vi "status_parser.vi"(4 "error in (no error)":errorcluster, 6 "Motor #":u8) -> (0 "error out":errorcluster, 1 "Program Complete?":bool, 2 "Motor # dup":u8)   [LabVIEW 2015]
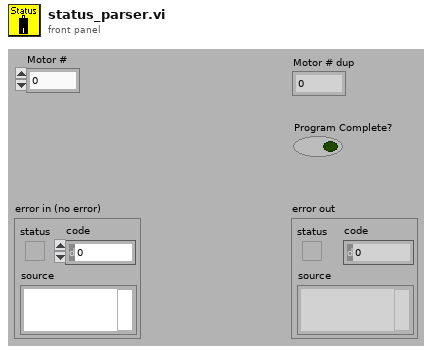
[diagram p1: front panel]
types:
  T1 = enum16{"POL (0)", "CPL (1)", "HLT (2)", "STP (3)", "RST (4)", "RVN (5)", "RPB (6)", "CLP (8)", "SDL (9)", "RUN (10)", "WRI (11)", "RRG (12)", "SPR (13)", "LPR (14)", "VMI (15)", "SSP (17)", "SSE (18)", "RIS (20)", "RIO (21)", "IMW (25)", "END (128)", "MAV (134)", "MRV (135)", "JRE (137)", "WCL (138)", "WCW (139)", "DLY (140)", "WDL (141)", "GCL (142)", "GOP (143)", "ZTG (144)", "ZTP (145)", "TTP (146)", "CME (147)", "CTC (148)", "TQL (149)", "AHC (150)", "ERL (151)", "OLP (152)", "WRP (154)", "IDT (155)", "LRP (156)", "VMP (159)", "RAV (160)", "RRV (161)", "JMP (162)", "JOI (162)", "CIS (163)", "CKS (164)", "CLC (165)", "KMC (167)", "MCT (168)", "FLC (169)", "EEM (170)", "DDB (171)", "DEM (171)", "PAC (172)", "ADL (173)", "BRT (174)", "MAT (176)", "MRT (177)", "RAT (178)", "RRT (179)", "SSD (180)", "KMR (181)", "KED (182)", "KDD (183)", "DIR (184)", "PRO (185)", "SIF (186)", "EDL (187)", "CIO (188)", "MDS (189)", "MDC (190)", "MDT (191)", "SEE (192)", "ARI (193)", "WBS (194)", "SCF (195)", "RSM (196)", "RLM (197)", "RSN (198)", "RLN (199)", "PCL (201)", "PCI (201)", "PRT (202)", "PRI (202)", "WBE (204)", "SOB (205)", "COB (206)", "ACR (207)", "PLR (208)", "CAI (211)", "LVT (212)", "OVT (213)", "MTT (214)", "CLC (215)", "PIM (216)", "VIM (217)", "TIM (218)", "AHM (219)", "SSL (221)", "TRU (222)", "RSD (223)", "EMT (225)", "DMT (226)", "EMD (227)", "DMD (228)", "HSM (229)", "AHD (230)", "PCM (231)", "PCG (232)", "XRV (233)", "XAV (234)", "XRT (235)", "XAT (236)", "GOC (237)", "JNA (238)", "JOR (239)", "PMC (240)", "PMV (241)", "PMX (242)", "DLC (243)", "SLC (244)", "PCP (245)", "ATR (248)", "PMO (249)", "JAN (250)", "EDH (251)", "DIF (252)", "IMS (253)", "IMQ (254)"}
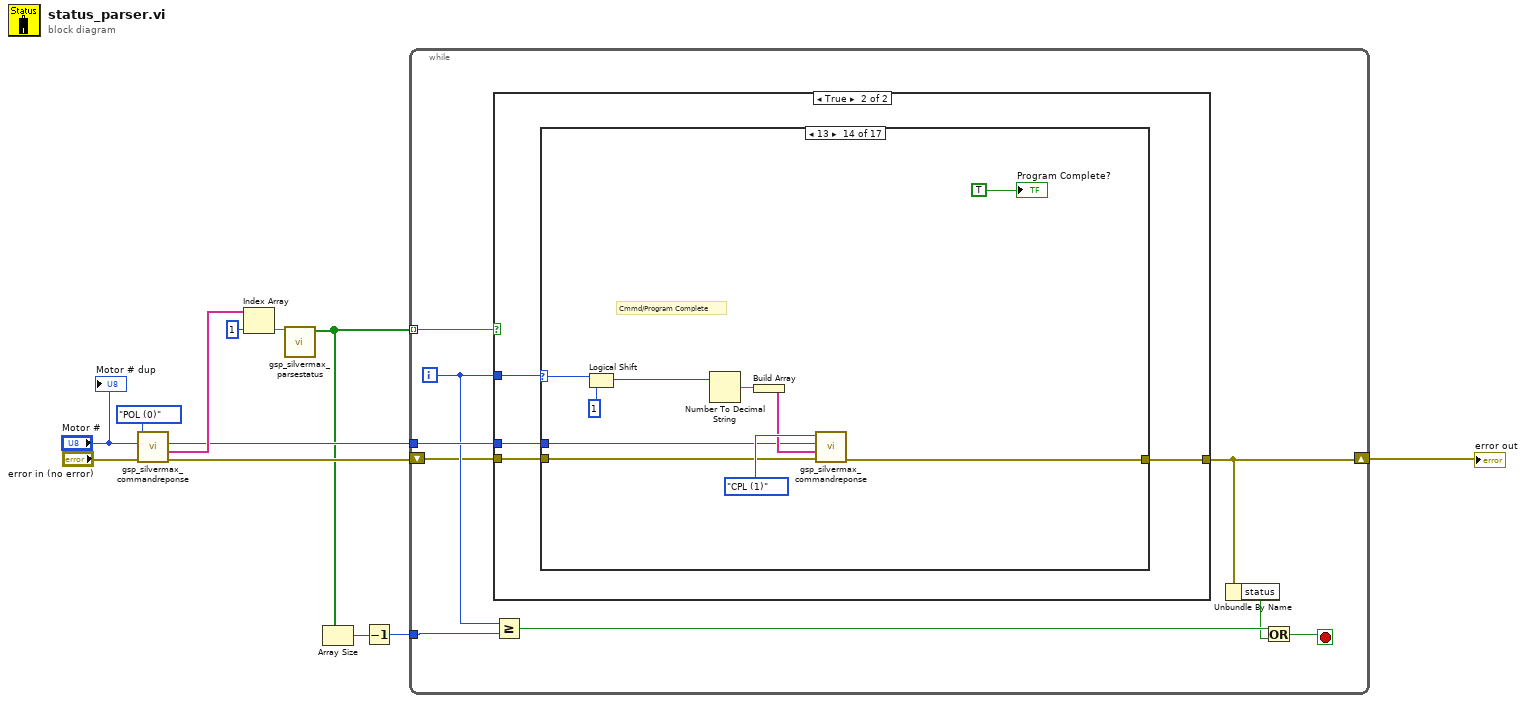
[diagram p0: block diagram]
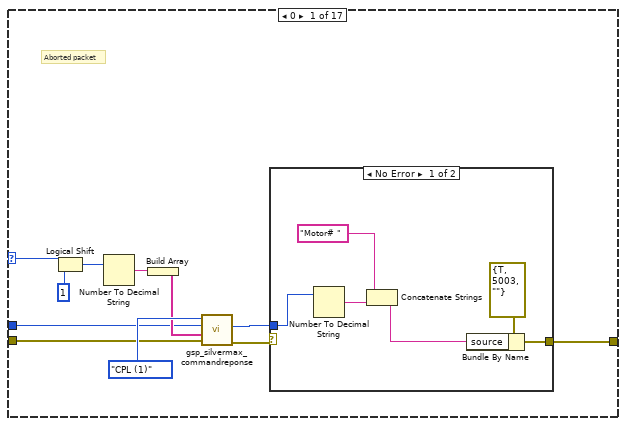
[diagram p3: hidden frame]
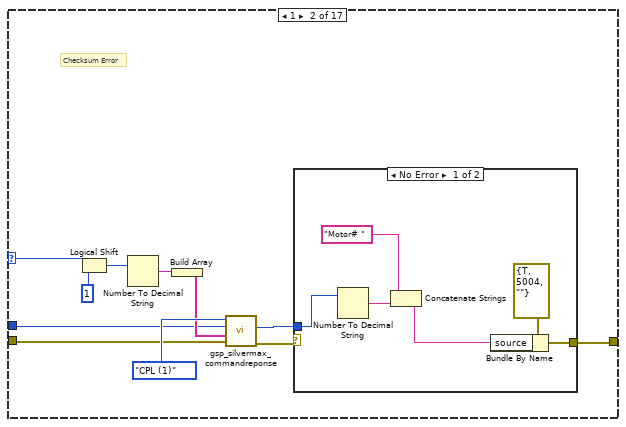
[diagram p5: hidden frame]
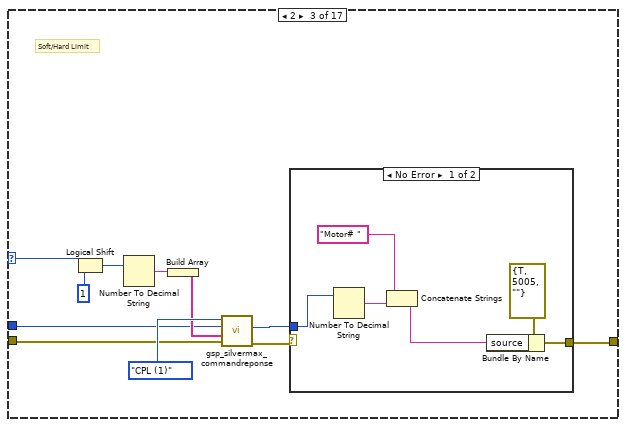
[diagram p7: hidden frame]
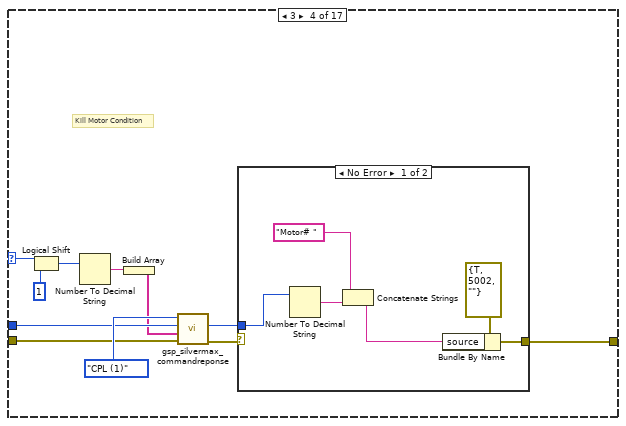
[diagram p9: hidden frame]
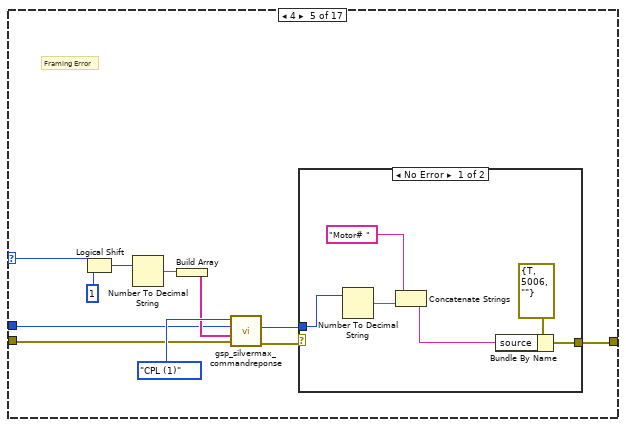
[diagram p11: hidden frame]
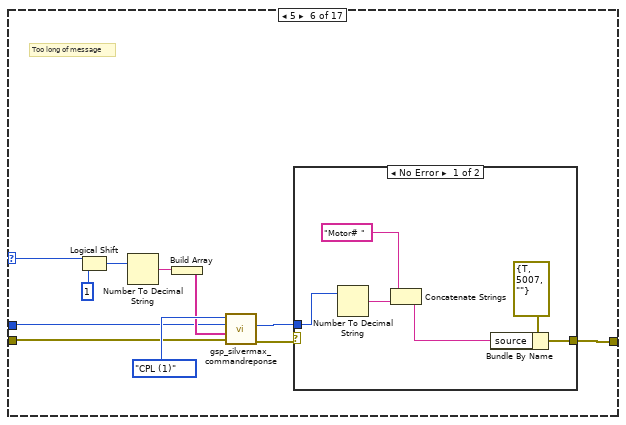
[diagram p13: hidden frame]
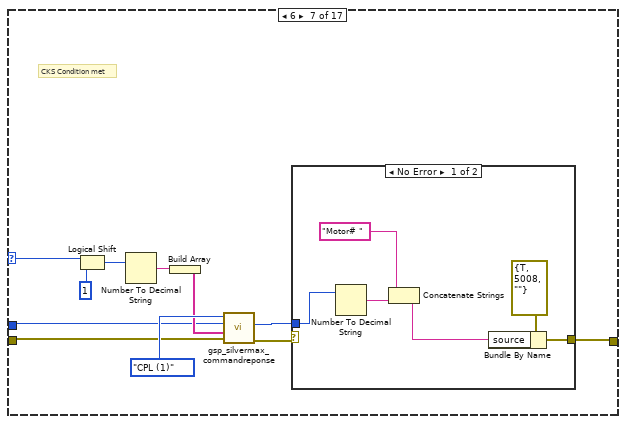
[diagram p15: hidden frame]
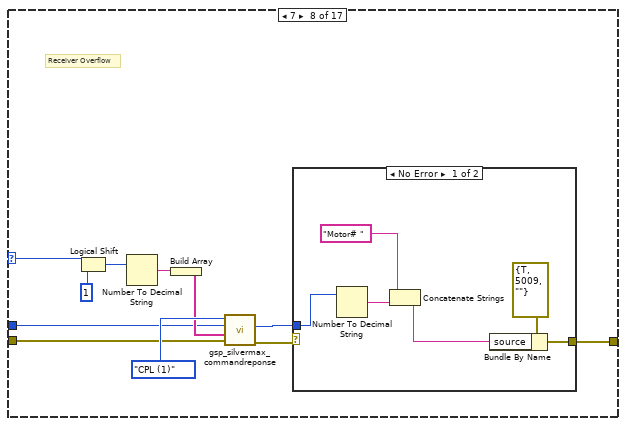
[diagram p17: hidden frame]
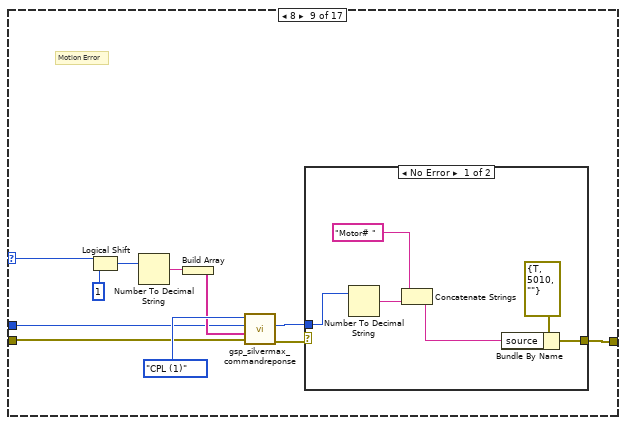
[diagram p19: hidden frame]
diagram:
  n1 = call "gsp_silvermax_commandreponse.vi"("error in (no error)"="error in (no error)", "Motor #"="Motor #", "Command"=T1."POL (0)") -> ("error out"=w8:errorcluster, "Parameter Array"=w9:string[], "Motor # dup"=w4:u8)  [unwired: 1 in, 1 out]
  n2 = Index Array(array=w9, index=1) -> (element=w10:string)
  n3 = call "gsp_silvermax_parsestatus.vi"("Status Word in Hex"=w10) -> ("Boolean Array"=w3:bool[])  [unwired: 6 in]
  n4 = Array Size(array=w3) -> (size(s)=w2:i32)
  n5 = Decrement(x=w2) -> (x-1=w1:i32)
  n6 = while {
    shift-right: [w14] -> w5
    shift-left: w8 -> [w16]
    tunnel: w3 -> [w21] mode=indexing
    tunnel: w4 -> [w20]
    tunnel: w1 -> [w18]
    i -> [w19]
    stop <- w15 stop-if-true
    n7 = case shown="True" w21 {
      tunnel: w19 -> [_ w26]
      tunnel: w16 -> [w22 w25]
      tunnel: [w22 w24] -> w14
      tunnel: w20 -> [_ w23]
      frame False {
      }
      frame True {
        n8 = case shown="13" w26 {
          selector: w26 -> [w28 w46 w63 w87 w100 w117 w135 w154 w171 w190 w207 _ w226 w252 w257 _ _]
          tunnel: w25 -> [w29 w48 w65 w89 w101 w119 w137 w156 w173 w191 w209 w225 w229 w247 w255 w272 w273]
          tunnel: [w27 w45 w64 w83 w99 w118 w136 w153 w174 w189 w208 w225 w227 w245 w254 w272 w273] -> w24
          tunnel: w23 -> [w30 w47 w66 w86 w102 w120 w138 w155 w172 w192 w210 _ w228 w246 w256 _ _]
          frame 0 {
            # "Aborted packet"
            n9 = Logical Shift(y=w28, x=u16 1) -> (x << y=w31:u16)
            n10 = Number To Decimal String(number=w31) -> (decimal integer string=w37:string)  [unwired: 1 in]
            n11 = Build Array(w37) -> (w34:string[])
            n12 = call "gsp_silvermax_commandreponse.vi"("error in (no error)"=w29, "Parameters (none)"=w34, "Motor #"=w30, "Command"=T1."CPL (1)") -> ("error out"=w33:errorcluster, "Motor # dup"=w32:u8)  [unwired: 2 out]
            n13 = case shown="No Error" w33 {
              selector: w33 -> [_ w44]
              tunnel: [w42 w44] -> w27
              tunnel: w32 -> [w40 _]
              frame No Error {
                n14 = Number To Decimal String(number=w40) -> (decimal integer string=w39:string)  [unwired: 1 in]
                n15 = Concatenate Strings("Motor# ", w39) -> (w38:string)
                n16 = Bundle By Name(cluster=errorcluster {"status"=TRUE, "code"=5003, "source"=""} ("error out"), "source"=w38) -> (w42:errorcluster)
              }
              frame Error {
              }
            }
          }
          frame 1 {
            # "Checksum Error"
            n17 = Logical Shift(y=w46, x=u16 1) -> (x << y=w49:u16)
            n18 = Number To Decimal String(number=w49) -> (decimal integer string=w55:string)  [unwired: 1 in]
            n19 = Build Array(w55) -> (w52:string[])
            n20 = call "gsp_silvermax_commandreponse.vi"("error in (no error)"=w48, "Parameters (none)"=w52, "Motor #"=w47, "Command"=T1."CPL (1)") -> ("error out"=w51:errorcluster, "Motor # dup"=w50:u8)  [unwired: 2 out]
            n21 = case shown="No Error" w51 {
              selector: w51 -> [_ w62]
              tunnel: [w60 w62] -> w45
              tunnel: w50 -> [w58 _]
              frame No Error {
                n22 = Number To Decimal String(number=w58) -> (decimal integer string=w57:string)  [unwired: 1 in]
                n23 = Concatenate Strings("Motor# ", w57) -> (w56:string)
                n24 = Bundle By Name(cluster=errorcluster {"status"=TRUE, "code"=5004, "source"=""} ("error out"), "source"=w56) -> (w60:errorcluster)
              }
              frame Error {
              }
            }
          }
          frame 2 {
            # "Soft/Hard Limit"
            n25 = Logical Shift(y=w63, x=u16 1) -> (x << y=w67:u16)
            n26 = Number To Decimal String(number=w67) -> (decimal integer string=w73:string)  [unwired: 1 in]
            n27 = Build Array(w73) -> (w70:string[])
            n28 = call "gsp_silvermax_commandreponse.vi"("error in (no error)"=w65, "Parameters (none)"=w70, "Motor #"=w66, "Command"=T1."CPL (1)") -> ("error out"=w69:errorcluster, "Motor # dup"=w68:u8)  [unwired: 2 out]
            n29 = case shown="No Error" w69 {
              selector: w69 -> [_ w80]
              tunnel: [w78 w80] -> w64
              tunnel: w68 -> [w76 _]
              frame No Error {
                n30 = Number To Decimal String(number=w76) -> (decimal integer string=w75:string)  [unwired: 1 in]
                n31 = Concatenate Strings("Motor# ", w75) -> (w74:string)
                n32 = Bundle By Name(cluster=errorcluster {"status"=TRUE, "code"=5005, "source"=""} ("error out"), "source"=w74) -> (w78:errorcluster)
              }
              frame Error {
              }
            }
          }
          frame 3 {
            # "Kill Motor Condition"
            n33 = Logical Shift(y=w87, x=u16 1) -> (x << y=w81:u16)
            n34 = Number To Decimal String(number=w81) -> (decimal integer string=w91:string)  [unwired: 1 in]
            n35 = Build Array(w91) -> (w85:string[])
            n36 = call "gsp_silvermax_commandreponse.vi"("error in (no error)"=w89, "Parameters (none)"=w85, "Motor #"=w86, "Command"=T1."CPL (1)") -> ("error out"=w84:errorcluster, "Motor # dup"=w82:u8)  [unwired: 2 out]
            n37 = case shown="No Error" w84 {
              selector: w84 -> [_ w98]
              tunnel: [w96 w98] -> w83
              tunnel: w82 -> [w94 _]
              frame No Error {
                n38 = Number To Decimal String(number=w94) -> (decimal integer string=w93:string)  [unwired: 1 in]
                n39 = Concatenate Strings("Motor# ", w93) -> (w92:string)
                n40 = Bundle By Name(cluster=errorcluster {"status"=TRUE, "code"=5002, "source"=""} ("error out"), "source"=w92) -> (w96:errorcluster)
              }
              frame Error {
              }
            }
          }
          frame 4 {
            # "Framing Error"
            n41 = Logical Shift(y=w100, x=u16 1) -> (x << y=w103:u16)
            n42 = Number To Decimal String(number=w103) -> (decimal integer string=w109:string)  [unwired: 1 in]
            n43 = Build Array(w109) -> (w106:string[])
            n44 = call "gsp_silvermax_commandreponse.vi"("error in (no error)"=w101, "Parameters (none)"=w106, "Motor #"=w102, "Command"=T1."CPL (1)") -> ("error out"=w105:errorcluster, "Motor # dup"=w104:u8)  [unwired: 2 out]
            n45 = case shown="No Error" w105 {
              selector: w105 -> [_ w116]
              tunnel: [w114 w116] -> w99
              tunnel: w104 -> [w112 _]
              frame No Error {
                n46 = Number To Decimal String(number=w112) -> (decimal integer string=w111:string)  [unwired: 1 in]
                n47 = Concatenate Strings("Motor# ", w111) -> (w110:string)
                n48 = Bundle By Name(cluster=errorcluster {"status"=TRUE, "code"=5006, "source"=""} ("error out"), "source"=w110) -> (w114:errorcluster)
              }
              frame Error {
              }
            }
          }
          frame 5 {
            # "Too long of message"
            n49 = Logical Shift(y=w117, x=u16 1) -> (x << y=w121:u16)
            n50 = Number To Decimal String(number=w121) -> (decimal integer string=w127:string)  [unwired: 1 in]
            n51 = Build Array(w127) -> (w124:string[])
            n52 = call "gsp_silvermax_commandreponse.vi"("error in (no error)"=w119, "Parameters (none)"=w124, "Motor #"=w120, "Command"=T1."CPL (1)") -> ("error out"=w123:errorcluster, "Motor # dup"=w122:u8)  [unwired: 2 out]
            n53 = case shown="No Error" w123 {
              selector: w123 -> [_ w134]
              tunnel: [w132 w134] -> w118
              tunnel: w122 -> [w130 _]
              frame No Error {
                n54 = Number To Decimal String(number=w130) -> (decimal integer string=w129:string)  [unwired: 1 in]
                n55 = Concatenate Strings("Motor# ", w129) -> (w128:string)
                n56 = Bundle By Name(cluster=errorcluster {"status"=TRUE, "code"=5007, "source"=""} ("error out"), "source"=w128) -> (w132:errorcluster)
              }
              frame Error {
              }
            }
          }
          frame 6 {
            # "CKS Condition met"
            n57 = Logical Shift(y=w135, x=u16 1) -> (x << y=w139:u16)
            n58 = Number To Decimal String(number=w139) -> (decimal integer string=w145:string)  [unwired: 1 in]
            n59 = Build Array(w145) -> (w142:string[])
            n60 = call "gsp_silvermax_commandreponse.vi"("error in (no error)"=w137, "Parameters (none)"=w142, "Motor #"=w138, "Command"=T1."CPL (1)") -> ("error out"=w141:errorcluster, "Motor # dup"=w140:u8)  [unwired: 2 out]
            n61 = case shown="No Error" w141 {
              selector: w141 -> [_ w152]
              tunnel: [w150 w152] -> w136
              tunnel: w140 -> [w148 _]
              frame No Error {
                n62 = Number To Decimal String(number=w148) -> (decimal integer string=w147:string)  [unwired: 1 in]
                n63 = Concatenate Strings("Motor# ", w147) -> (w146:string)
                n64 = Bundle By Name(cluster=errorcluster {"status"=TRUE, "code"=5008, "source"=""} ("error out"), "source"=w146) -> (w150:errorcluster)
              }
              frame Error {
              }
            }
          }
          frame 7 {
            # "Receiver Overflow"
            n65 = Logical Shift(y=w154, x=u16 1) -> (x << y=w157:u16)
            n66 = Number To Decimal String(number=w157) -> (decimal integer string=w163:string)  [unwired: 1 in]
            n67 = Build Array(w163) -> (w160:string[])
            n68 = call "gsp_silvermax_commandreponse.vi"("error in (no error)"=w156, "Parameters (none)"=w160, "Motor #"=w155, "Command"=T1."CPL (1)") -> ("error out"=w159:errorcluster, "Motor # dup"=w158:u8)  [unwired: 2 out]
            n69 = case shown="No Error" w159 {
              selector: w159 -> [_ w170]
              tunnel: [w168 w170] -> w153
              tunnel: w158 -> [w166 _]
              frame No Error {
                n70 = Number To Decimal String(number=w166) -> (decimal integer string=w165:string)  [unwired: 1 in]
                n71 = Concatenate Strings("Motor# ", w165) -> (w164:string)
                n72 = Bundle By Name(cluster=errorcluster {"status"=TRUE, "code"=5009, "source"=""} ("error out"), "source"=w164) -> (w168:errorcluster)
              }
              frame Error {
              }
            }
          }
          frame 8 {
            # "Motion Error"
            n73 = Logical Shift(y=w171, x=u16 1) -> (x << y=w175:u16)
            n74 = Number To Decimal String(number=w175) -> (decimal integer string=w181:string)  [unwired: 1 in]
            n75 = Build Array(w181) -> (w178:string[])
            n76 = call "gsp_silvermax_commandreponse.vi"("error in (no error)"=w173, "Parameters (none)"=w178, "Motor #"=w172, "Command"=T1."CPL (1)") -> ("error out"=w177:errorcluster, "Motor # dup"=w176:u8)  [unwired: 2 out]
            n77 = case shown="No Error" w177 {
              selector: w177 -> [_ w188]
              tunnel: [w186 w188] -> w174
              tunnel: w176 -> [w184 _]
              frame No Error {
                n78 = Number To Decimal String(number=w184) -> (decimal integer string=w183:string)  [unwired: 1 in]
                n79 = Concatenate Strings("Motor# ", w183) -> (w182:string)
                n80 = Bundle By Name(cluster=errorcluster {"status"=TRUE, "code"=5010, "source"=""} ("error out"), "source"=w182) -> (w186:errorcluster)
              }
              frame Error {
              }
            }
          }
          frame 9 {
            # "Holding Error"
            n81 = Logical Shift(y=w190, x=u16 1) -> (x << y=w193:u16)
            n82 = Number To Decimal String(number=w193) -> (decimal integer string=w199:string)  [unwired: 1 in]
            n83 = Build Array(w199) -> (w196:string[])
            n84 = call "gsp_silvermax_commandreponse.vi"("error in (no error)"=w191, "Parameters (none)"=w196, "Motor #"=w192, "Command"=T1."CPL (1)") -> ("error out"=w195:errorcluster, "Motor # dup"=w194:u8)  [unwired: 2 out]
            n85 = case shown="No Error" w195 {
              selector: w195 -> [_ w206]
              tunnel: [w204 w206] -> w189
              tunnel: w194 -> [w202 _]
              frame No Error {
                n86 = Number To Decimal String(number=w202) -> (decimal integer string=w201:string)  [unwired: 1 in]
                n87 = Concatenate Strings("Motor# ", w201) -> (w200:string)
                n88 = Bundle By Name(cluster=errorcluster {"status"=TRUE, "code"=5011, "source"=""} ("error out"), "source"=w200) -> (w204:errorcluster)
              }
              frame Error {
              }
            }
          }
          frame 10 {
            # "Low/Over Voltage"
            n89 = Logical Shift(y=w207, x=u16 1) -> (x << y=w211:u16)
            n90 = Number To Decimal String(number=w211) -> (decimal integer string=w217:string)  [unwired: 1 in]
            n91 = Build Array(w217) -> (w214:string[])
            n92 = call "gsp_silvermax_commandreponse.vi"("error in (no error)"=w209, "Parameters (none)"=w214, "Motor #"=w210, "Command"=T1."CPL (1)") -> ("error out"=w213:errorcluster, "Motor # dup"=w212:u8)  [unwired: 2 out]
            n93 = case shown="No Error" w213 {
              selector: w213 -> [_ w224]
              tunnel: [w222 w224] -> w208
              tunnel: w212 -> [w220 _]
              frame No Error {
                n94 = Number To Decimal String(number=w220) -> (decimal integer string=w219:string)  [unwired: 1 in]
                n95 = Concatenate Strings("Motor# ", w219) -> (w218:string)
                n96 = Bundle By Name(cluster=errorcluster {"status"=TRUE, "code"=5012, "source"=""} ("error out"), "source"=w218) -> (w222:errorcluster)
              }
              frame Error {
              }
            }
          }
          frame 11 {
            # "Move Terminated with Sensor found"
          }
          frame 12 {
            # "Command Error"
            n97 = Logical Shift(y=w226, x=u16 1) -> (x << y=w230:u16)
            n98 = Number To Decimal String(number=w230) -> (decimal integer string=w236:string)  [unwired: 1 in]
            n99 = Build Array(w236) -> (w233:string[])
            n100 = call "gsp_silvermax_commandreponse.vi"("error in (no error)"=w229, "Parameters (none)"=w233, "Motor #"=w228, "Command"=T1."CPL (1)") -> ("error out"=w232:errorcluster, "Motor # dup"=w231:u8)  [unwired: 2 out]
            n101 = case shown="No Error" w232 {
              selector: w232 -> [_ w243]
              tunnel: [w241 w243] -> w227
              tunnel: w231 -> [w239 _]
              frame No Error {
                n102 = Number To Decimal String(number=w239) -> (decimal integer string=w238:string)  [unwired: 1 in]
                n103 = Concatenate Strings("Motor# ", w238) -> (w237:string)
                n104 = Bundle By Name(cluster=errorcluster {"status"=TRUE, "code"=5014, "source"=""} ("error out"), "source"=w237) -> (w241:errorcluster)
              }
              frame Error {
              }
            }
          }
          frame 13 {
            # "Cmmd/Program Complete"
            n105 = Logical Shift(y=w252, x=u16 1) -> (x << y=w244:u16)
            n106 = Number To Decimal String(number=w244) -> (decimal integer string=w250:string)  [unwired: 1 in]
            n107 = Build Array(w250) -> (w248:string[])
            n108 = call "gsp_silvermax_commandreponse.vi"("error in (no error)"=w247, "Parameters (none)"=w248, "Motor #"=w246, "Command"=T1."CPL (1)") -> ("error out"=w245:errorcluster)  [unwired: 3 out]
            "Program Complete?" <- TRUE
          }
          frame 14 {
            # "NVM Checksum Error"
            n109 = Logical Shift(y=w257, x=u16 1) -> (x << y=w258:u16)
            n110 = Number To Decimal String(number=w258) -> (decimal integer string=w264:string)  [unwired: 1 in]
            n111 = Build Array(w264) -> (w261:string[])
            n112 = call "gsp_silvermax_commandreponse.vi"("error in (no error)"=w255, "Parameters (none)"=w261, "Motor #"=w256, "Command"=T1."CPL (1)") -> ("error out"=w260:errorcluster, "Motor # dup"=w259:u8)  [unwired: 2 out]
            n113 = case shown="No Error" w260 {
              selector: w260 -> [_ w271]
              tunnel: [w269 w271] -> w254
              tunnel: w259 -> [w267 _]
              frame No Error {
                n114 = Number To Decimal String(number=w267) -> (decimal integer string=w266:string)  [unwired: 1 in]
                n115 = Concatenate Strings("Motor# ", w266) -> (w265:string)
                n116 = Bundle By Name(cluster=errorcluster {"status"=TRUE, "code"=5015, "source"=""} ("error out"), "source"=w265) -> (w269:errorcluster)
              }
              frame Error {
              }
            }
          }
          frame 15 {
            # "Foreground Command Done"
          }
          frame 16, Default {
          }
        }
      }
    }
    n117 = Greater Or Equal?(x=w19, y=w18) -> (x >= y?=w17:bool)
    n118 = Unbundle By Name(w14) -> ("status"=w13:bool)
    n119 = Or(x=w17, y=w13) -> (x .or. y?=w15:bool)
  }
  "error out" <- w5
  "Motor # dup" <- "Motor #"
